vi "SetDACAlltozero.vi"(1 "All to zero":bool=TRUE, 2 "DAC write (mV)":dbl[](array[numeric]) min=-2000.0 max=2000.0, 3 "RS232/ Optical Fiber":refnum<visa-resource-name>="COM4") -> (0 "DAC read (mV)":dbl[](array[numeric]))   [LabVIEW 2011]
uses:
  Visa name1.vi
panel:
  # "old Cryofree: COM4"
  # "Set dac value manually\nDac values are swept safely"
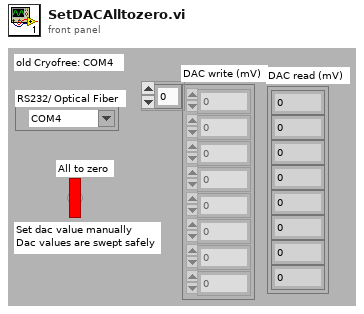
[diagram p1: front panel]
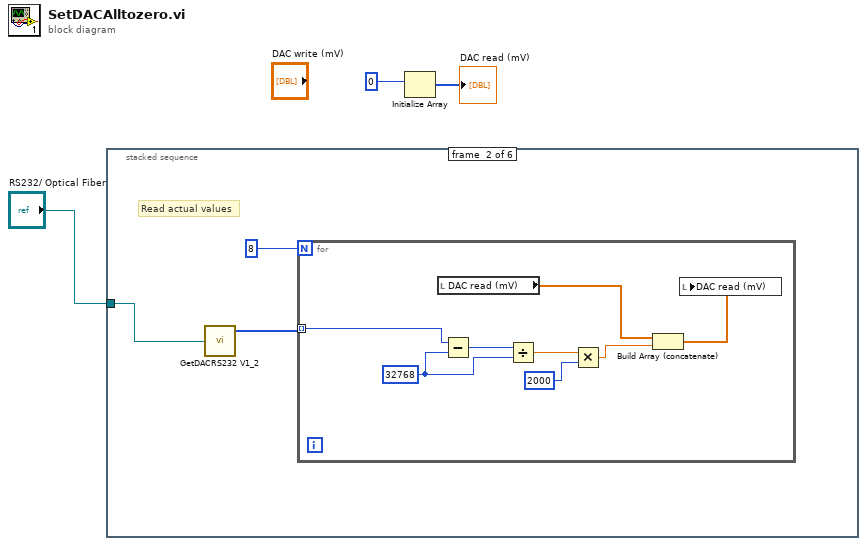
[diagram p0: block diagram]
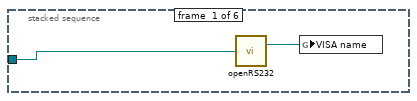
[diagram p2: hidden frame]
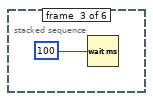
[diagram p3: hidden frame]
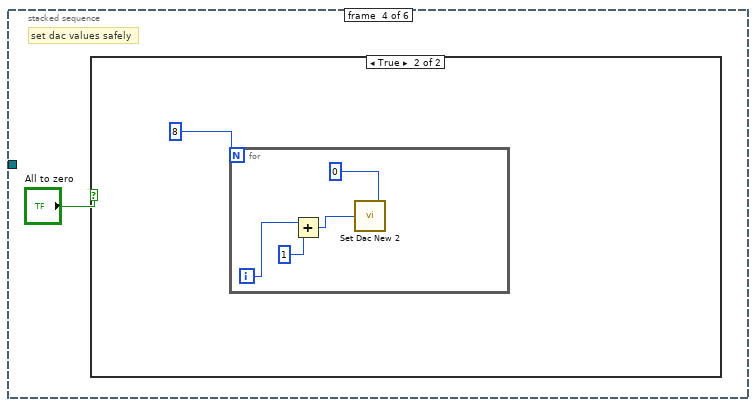
[diagram p4: hidden frame]
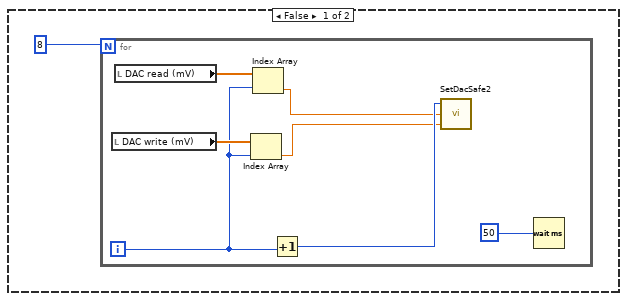
[diagram p5: hidden frame]
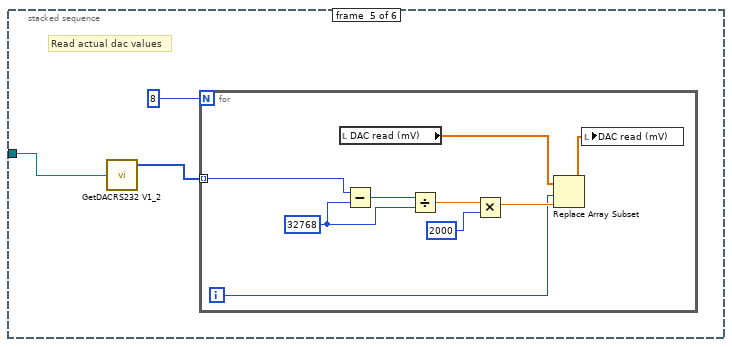
[diagram p6: hidden frame]
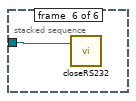
[diagram p7: hidden frame]
diagram:
  n1 = stacked-sequence {
    tunnel: "RS232/ Optical Fiber" -> [w5 w8 _ _ w34 w44]
    frame #0 {
      n2 = call "openRS232.vi"("com"=w5) -> ("VISA resource name"=w4:refnum<visa-resource-name>)  [unwired: 1 out]
      n3 = global write "Visa name1.vi" "VISA name"(w4) -> ()
    }
    frame #1 {
      # "Read actual values"
      n4 = call "GetDACRS232 V1_2.vi"("VISA resource name IN"=w8) -> ("DAC data out\n(hexadecimaal)"=w6:u16[])  [unwired: 2 in, 2 out]
      n5 = for {
        N: 8 -> [_]
        tunnel: w6 -> [w12] mode=indexing
        w15 = 32768
        n6 = local read "DAC read (mV)"() -> (w11:dbl[])
        n7 = Subtract(x=w12, y=w15) -> (x-y=w16:i32)
        n8 = Divide(x=w16, y=w15) -> (x/y=w14:dbl)
        n9 = Multiply(x=w14, y=2000) -> (x*y=w9:dbl)
        n10 = Build Array (concatenate)(w11, w9) -> (w10:dbl[])
        n11 = local write "DAC read (mV)"(w10) -> ()
      }
    }
    frame #2 {
      n12 = Wait (ms)(milliseconds to wait=100) -> ()  [unwired: 1 out]
    }
    frame #3 {
      # "set dac values safely"
      n13 = case shown="True" "All to zero" {
        frame False {
          n14 = for {
            N: 8 -> [_]
            i -> [w23]
            n15 = local read "DAC write (mV)"() -> (w25:dbl[])
            n16 = local read "DAC read (mV)"() -> (w24:dbl[])
            n17 = Index Array(array=w25, index=w23) -> (element=w22:dbl)
            n18 = Index Array(array=w24, index=w23) -> (element=w21:dbl)
            n19 = Increment(x=w23) -> (x+1=w26:i32)
            n20 = call "SetDacSafe2.vi"("New Value (mV)"=w22, "Actual Value DAC (mV)"=w21, "DAC Nr."=w26) -> ()  [unwired: 1 out]
            n21 = Wait (ms)(milliseconds to wait=50) -> ()  [unwired: 1 out]
          }
        }
        frame True {
          n22 = for {
            N: 8 -> [_]
            i -> [w30]
            n23 = Add(x=w30, y=1) -> (x+y=w29:i32)
            n24 = call "Set Dac New 2.vi"("DATA (V)"=0, "DAC nr"=w29) -> ()
          }
        }
      }
    }
    frame #4 {
      # "Read actual dac values"
      n25 = call "GetDACRS232 V1_2.vi"("VISA resource name IN"=w34) -> ("DAC data out\n(hexadecimaal)"=w32:u16[])  [unwired: 2 in, 2 out]
      n26 = for {
        N: 8 -> [_]
        tunnel: w32 -> [w39] mode=indexing
        i -> [w35]
        w42 = 32768
        n27 = local read "DAC read (mV)"() -> (w38:dbl[])
        n28 = Subtract(x=w39, y=w42) -> (x-y=w43:i32)
        n29 = Divide(x=w43, y=w42) -> (x/y=w41:dbl)
        n30 = Multiply(x=w41, y=2000) -> (x*y=w36:dbl)
        n31 = Replace Array Subset(array=w38, new element=w36, index=w35) -> (w37:dbl[])
        n32 = local write "DAC read (mV)"(w37) -> ()
      }
    }
    frame #5 {
      n33 = call "closeRS232.vi"("VISA resource name"=w44) -> ()  [unwired: 2 in]
    }
  }
  n34 = Initialize Array(0) -> (→"DAC read (mV)":i32[])  [unwired: 1 in]
